vi "BotSpeakSerial_WriteRead.vi"(0 "error In":errorcluster, 1 "To Write":string, 2 "Bot Settings in":T1) -> (3 "error out":errorcluster, 4 "Reply":string, 5 "Reply EOF":string, 6 "Bot Settings out":T1)   [LabVIEW 2012]
uses:
  <userlib>/botspeak/VIs/Direct/BotSpeak_Control.ctl
  <userlib>/botspeak/VIs/SubVIs/BotSpeak_Globals.vi
panel:
  out "iterations":i32
  out "Buffer":u32[](graph)
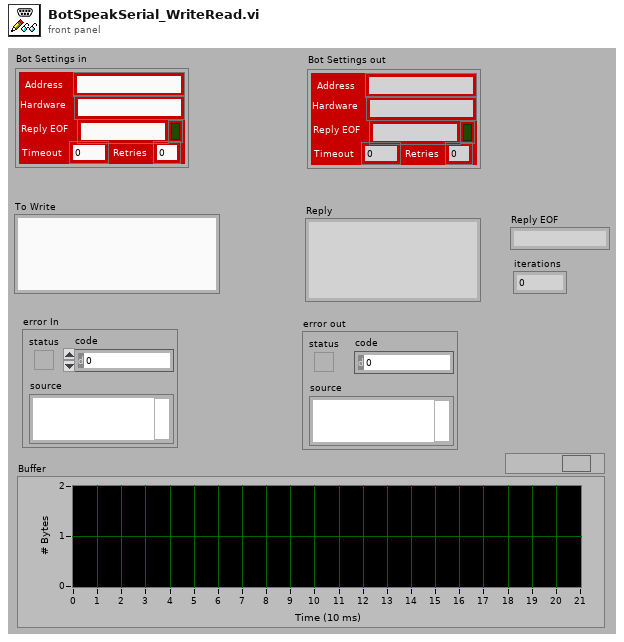
[diagram p1: front panel]
types:
  T1 = typedef "BotSpeak_Control.ctl" = cluster{"Address":string, "Reply EOF":string, "Hardware":string, "Retries":i8, "Timeout":i32, "Open?":bool}
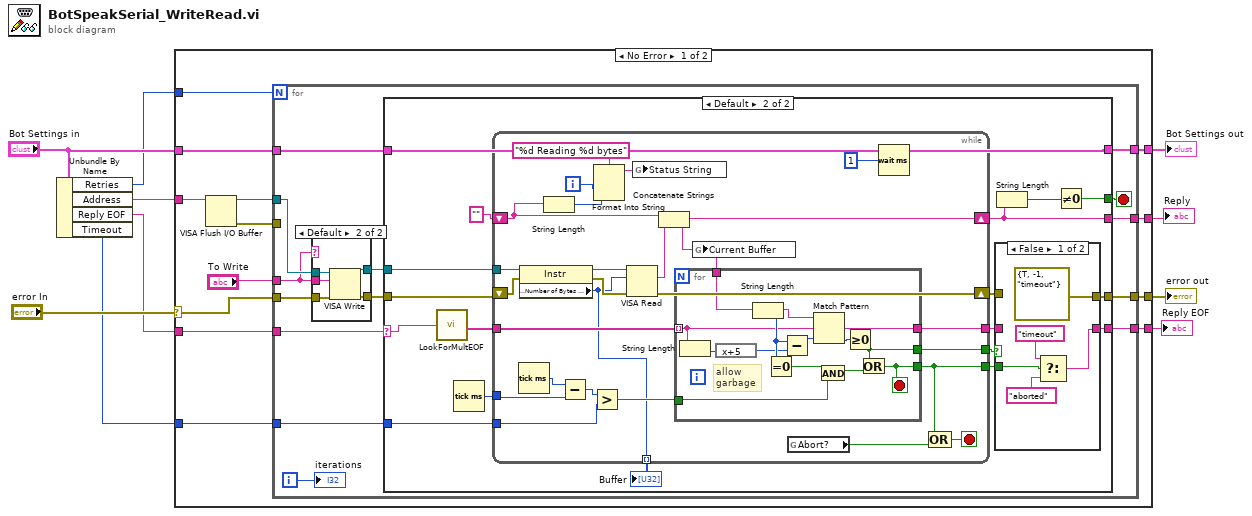
[diagram p0: block diagram]
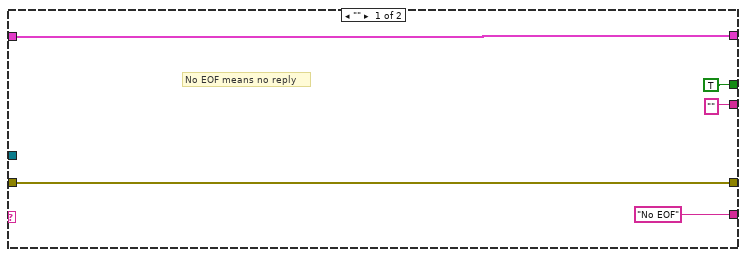
[diagram p3: hidden frame]
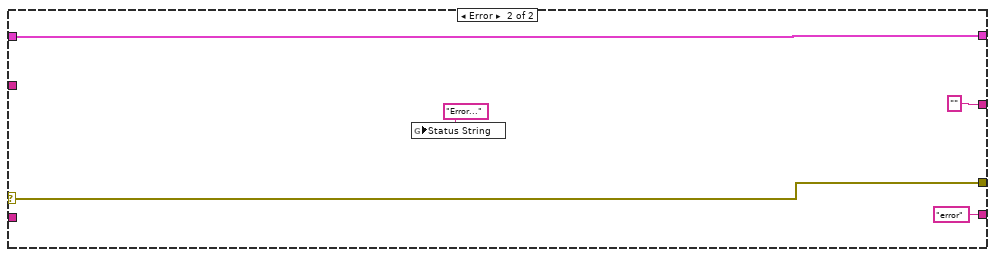
[diagram p5: hidden frame]
diagram:
  n1 = Unbundle By Name("Bot Settings in") -> ("Retries"=w4:i8, "Address"=w5:string, "Reply EOF"=w2:string, "Timeout"=w3:i32)
  n2 = case shown="No Error" "error In" {
    selector: "error In" -> [w15 w114]
    tunnel: [w23 ""] -> w7
    tunnel: [w22 w114] -> w8
    tunnel: "Bot Settings in" -> [w21 w112]
    tunnel: [w20 w112] -> w9
    tunnel: w4 -> [w19 _]
    tunnel: w5 -> [w13 _]
    tunnel: w3 -> [w18 _]
    tunnel: w2 -> [w16 _]
    tunnel: [w14 "error" ("Reply EOF")] -> w1
    frame No Error {
      n3 = VISA Flush I/O Buffer(VISA resource name=w13) -> (VISA resource name out=w11:refnum<visa-resource-name>, error out=w12:errorcluster)  [unwired: 2 in]
      n4 = for {
        N: w19 -> [_]
        tunnel: "To Write" -> [w25]
        tunnel: [w37] -> w23
        tunnel: [w32] -> w22
        tunnel: w15 -> [w36]
        tunnel: w21 -> [w30]
        tunnel: [w33] -> w20
        tunnel: w18 -> [w29]
        tunnel: w16 -> [w28]
        tunnel: w11 -> [w27]
        tunnel: [w26] -> w14
        tunnel: w12 -> [_]
        i -> [w24]
        stop <- w31 stop-if-true
        n5 = case shown="Default" w25 {
          tunnel: w25 -> [_ w44]
          tunnel: w36 -> [w39 w43]
          tunnel: [w38 w42] -> w35
          tunnel: [w39 w41] -> w34
          tunnel: w27 -> [w38 w40]
          frame "" {
          }
          frame Default {
            n6 = VISA Write(VISA resource name=w40, write buffer=w44, error in (no error)=w43) -> (VISA resource name out=w42:refnum<visa-resource-name>, error out=w41:errorcluster)  [unwired: 1 out]
          }
        }
        n7 = case shown="Default" w28 {
          selector: w28 -> [_ w53]
          tunnel: ["" w63] -> w37
          tunnel: [w48 w51] -> w32
          tunnel: w35 -> [_ w66]
          tunnel: w34 -> [w48 w65]
          tunnel: w30 -> [w45 w52]
          tunnel: [w45 w52] -> w33
          tunnel: [TRUE w55] -> w31
          tunnel: w29 -> [_ w61]
          tunnel: ["No EOF" ("Reply EOF") w57] -> w26
          frame "" {
            # "No EOF means no reply"
          }
          frame Default {
            n8 = call <userlib>:"LookForMultEOF.vi"("Reply EOF"=w53) -> ("Array"=w60:string[])
            n9 = Tick Count (ms)() -> (millisecond timer value=w64:u32)
            n10 = while {
              tunnel: w60 -> [w94]
              shift-right: [w99] -> w50
              shift-left: w65 -> [w98]
              shift-right: [w81] -> w63
              shift-left: "" -> [w84]
              tunnel: w66 -> [w93]
              tunnel: w64 -> [w88]
              tunnel: w61 -> [w79]
              tunnel: [w77] -> w59
              tunnel: [w78] -> w58
              tunnel: [w76] -> w56
              tunnel: [w75] -> w54 mode=indexing
              i -> [w86]
              stop <- w90 stop-if-true
              n11 = Tick Count (ms)() -> (millisecond timer value=w89:u32)
              n12 = property class="Instr"(reference=w93, error in=w98) -> (reference out=w97:refnum<visa-resource-name>, error out=w96:errorcluster, "Serial Settings:Number of Bytes at Serial Port"=w75:u32)
              n13 = String Length(string=w84) -> (length=w83:i32)
              n14 = Subtract(x=w89, y=w88) -> (x-y=w92:u32)
              n15 = Greater?(x=w92, y=w79) -> (0:w91:bool)
              n16 = Format Into String(format string="%d Reading %d bytes", w86, w83) -> (resulting string=w85:string)  [unwired: 2 in, 1 out]
              n17 = VISA Read(VISA resource name=w97, byte count=w75, error in (no error)=w96) -> (read buffer=w95:string, error out=w99:errorcluster)  [unwired: 2 out]
              n18 = global write "BotSpeak_Globals.vi" "Status String"(w85) -> ()
              n19 = Concatenate Strings(w84, w95) -> (w81:string)
              n20 = for {
                tunnel: w94 -> [w103] mode=indexing
                tunnel: w91 -> [w110]
                tunnel: w81 -> [w101]
                tunnel: [w104] -> w76
                tunnel: [w103] -> w78
                tunnel: [w102] -> w77
                stop <- w104 stop-if-true
                # "allow\ngarbage"
                n21 = String Length(string=w103) -> (length=w108:i32)
                n22 = expression code="x+5"(w108) -> (w100:i32)
                n23 = String Length(string=w101) -> (length=w106:i32)
                n24 = Equal To 0?(x=w106) -> (x = 0?=w109:bool)
                n25 = Subtract(x=w106, y=w100) -> (x-y=w107:i32)
                n26 = Match Pattern(string=w101, regular expression=w103, offset (0)=w107) -> (offset past match=w111:i32)  [unwired: 3 out]
                n27 = And(x=w109, y=w110) -> (x .and. y?=w105:bool)
                n28 = Greater Or Equal To 0?(x=w111) -> (x >= 0?=w102:bool)
                n29 = Or(x=w102, y=w105) -> (x .or. y?=w104:bool)
              }
              n30 = global write "BotSpeak_Globals.vi" "Current Buffer"(w81) -> ()
              n31 = global read "BotSpeak_Globals.vi" "Abort?"() -> (w80:bool)
              n32 = Wait (ms)(milliseconds to wait=u32 1) -> ()  [unwired: 1 out]
              n33 = Compound Arithmetic op=OR(w76, w80) -> (w90:bool)
            }
            "Buffer" <- w54
            n34 = case shown="False" w59 {
              tunnel: w58 -> [_ w74]
              tunnel: [w69 w74] -> w57
              tunnel: w56 -> [w71 _]
              tunnel: [errorcluster {"status"=TRUE, "code"=-1, "source"="timeout"} ("error out") w73] -> w51
              tunnel: w50 -> [_ w73]
              frame False {
                n35 = Select(t="timeout" ("Reply EOF"), s=w71, f="aborted" ("Reply EOF")) -> (s? t:f=w69:string)
              }
              frame True {
              }
            }
            n36 = String Length(string=w63) -> (length=w62:i32)
            n37 = Not Equal To 0?(x=w62) -> (x != 0?=w55:bool)
          }
        }
        "iterations" <- w24
      }
    }
    frame Error {
      n38 = global write "BotSpeak_Globals.vi" "Status String"("Error..." ("Status String")) -> ()
    }
  }
  "Bot Settings out" <- w9
  "error out" <- w8
  "Reply" <- w7
  "Reply EOF" <- w1
